vi "SlowLogger_Close.vi"(8 "error in (no error)":errorcluster, 11 "SlowLogger in":refnum<class "SlowLogger.lvclass">) -> (0 "error out":errorcluster)   [LabVIEW 2018, in "feGEM DataPacker.lvlib" / "SlowLogger.lvclass"]
uses:
  SlowLogger.lvclass
  SlowLogger.lvclass/SlowLogger.ctl
panel:
  out "Remaining elements in queue after close":i32
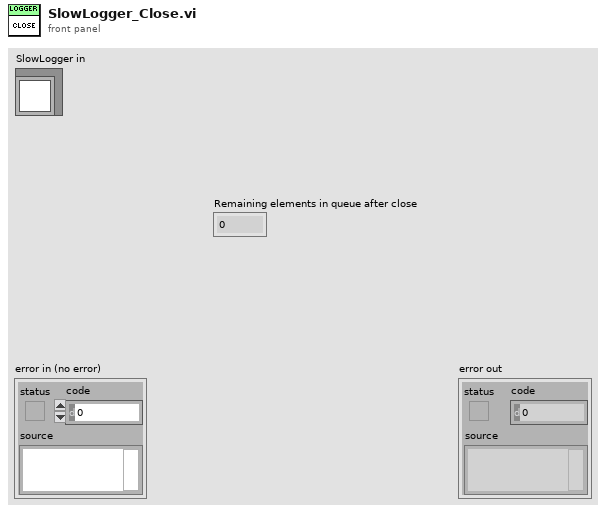
[diagram p1: front panel]
types:
  T1 = typedef "feGEM DataPacker.lvlib/GEM_BANK_CLUSTER_typedef.ctl" = cluster{"Category":string, "Variable Name":string, "Equipment description":string, "History Settings":u16, "Period to update history plots":u16, "GEM_DATA Cluster":T2}
  T2 = typedef "feGEM DataPacker.lvlib/GEM_DATA_cluster_typedef.ctl" = cluster{"DataType":string, "Formatted Data":u8[], "data byte order (Little Endian prefered)":enum16{"big-endian, network order", "native, host order", "little-endian"}}
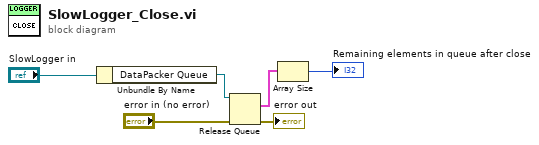
[diagram p0: block diagram]
diagram:
  n1 = Unbundle By Name("SlowLogger in") -> ("DataPacker Queue"=w2:refnum<queue>)
  n2 = Release Queue(queue=w2, error in (no error)="error in (no error)") -> (remaining elements=w1:T1[], error out=→"error out":errorcluster)  [unwired: 1 in, 1 out]
  n3 = Array Size(array=w1) -> (size(s)=→"Remaining elements in queue after close":i32)
